vi "TURCK GUI TestPanel alle Module Test Lampe.vi"() -> ()   [LabVIEW 2017]
doc: "Example for reading and writing values for the TBEN-S2-2RFID-4DXP module from Turck"
uses:
  KH TURCK ETHERNETIP TDef Enum RFID Error.ctl
  KH TURCK ETHERNETIP TDefCluster TBEN-S2-2RFID-4DXP Status.ctl
  KH EthernetIPConfig 17.14/KH EthernetIPConfig TDef Config.ctl
  KH EthernetIPConfig 17.14/KH EthernetIPConfig TypeDefs ModuleTyp.ctl
  KH_DAQ 17.04/Turck/KH_DAQ_TURCK_TypeDefs_Cluster DI.ctl
  KH_DAQ 17.04/KH_DAQ_TypeDefs_Cluster AO.ctl
  KH_DAQ 17.04/KH_DAQ_TypeDefs_Messbereich.ctl
  KH_DAQ 17.04/KH_DAQ_TypeDefs_Bereich.ctl
  KH_DAQ 17.04/KH_DAQ_TypeDefs_Cluster AI.ctl
  KH TURCK ETHERNETIP TDef Enum IOL Data.ctl
  KH_DAQ 17.04/Turck/KH_DAQ_TURCK_TypeDefs_Cluster DO.ctl
  KH TURCK ETHERNETIP TDef Enum RFID Data RFID.ctl
  KH TURCK TypeDefs FGlob.ctl
  KH TURCK ETHERNETIP TDef Enum RFID User Command.ctl
  KH EthernetIP 17.19/KH_EthernetIP_Globals.vi
  KH TURCK ETHERNETIP RFID Global.vi
  KH TURCK ETHERNETIP RFID ST READ Global.vi
  KH TURCK ETHERNETIP Global.vi
panel:
  in  "Reset 7":bool
  in  "Reset 6":bool
  in  "Reset 5":bool
  in  "Reset 4":bool
  in  "Reset 3":bool
  in  "Reset 2":bool
  in  "Reset 1":bool
  in  "Reset 0":bool
  in  "Signal Name":string[](array[string])=["IOL1", "IOL3", "ARFID2", "ARFID3", "BRFID0", "BRFID1", "ADXP0", "ADXP2", "ADXP6", "ADXP7", "BDXP1", "BDXP2", "BDXP3", "BDXP7"]
  in  "DI":string[](array[string])=["IOL0", "IOL2", "ARFID0", "ARFID1", "BRFID2", "BRFID3", "ADXP1", "ADXP3", "ADXP4", "ADXP5", "BDXP0", "BDXP4", "BDXP5", "BDXP6"]
  out "DO in":bool[](array[boolean])
  out "DI":bool[](array[boolean])
  in  "AO Values":sgl[](array[numeric])=[0.0, 0.0, 0.0, 0.0, 0.0, 0.0, 0.0, 0.0] format="%.6f"
  in  "DO":bool[](array[boolean])=[FALSE, FALSE, FALSE, FALSE, FALSE, FALSE, FALSE, FALSE, FALSE, FALSE, FALSE, FALSE, FALSE, FALSE]
  in  "Tab Control":T1(tab)
  in  "EIP_DO":T2={"Def"=[], "Signal Name"=["IOL1", "IOL3", "ARFID2", "ARFID3", "BRFID0", "BRFID1", "ADXP0", "ADXP2", "ADXP6", "ADXP7", "BDXP1", "BDXP2", "BDXP3", "BDXP7"], "Description"=[], "Chan"=[], "Inv"=[], "Nr"=[1, 1, 1, 1, 2, 2, 1, 1, 1, 1, 2, 2, 2, 2], "SensorType"=[enum."TBEN-S2-4IOL", enum."TBEN-S2-4IOL", enum."TBEN-S2-2RFID-4DXP", enum."TBEN-S2-2RFID-4DXP", enum."TBEN-S2-2RFID-4DXP", enum."TBEN-S2-2RFID-4DXP", enum."TBEN-S1-8DXP", enum."TBEN-S1-8DXP", enum."TBEN-S1-8DXP", enum."TBEN-S1-8DXP", enum."TBEN-S1-8DXP", enum."TBEN-S1-8DXP", enum."TBEN-S1-8DXP", enum."TBEN-S1-8DXP"]} {"Nr" max=63; "Chan" max=63}
  in  "EIP_DI":T4={"Signal Name"=["IOL0", "IOL2", "ARFID0", "ARFID1", "BRFID2", "BRFID3", "ADXP1", "ADXP3", "ADXP4", "ADXP5", "BDXP0", "BDXP4", "BDXP5", "BDXP6"], "Description"=[], "Chan"=[], "Inv"=[], "Nr"=[1, 1, 1, 1, 2, 2, 1, 1, 1, 1, 2, 2, 2, 2], "SensorType"=[enum."TBEN-S2-4IOL", enum."TBEN-S2-4IOL", enum."TBEN-S2-2RFID-4DXP", enum."TBEN-S2-2RFID-4DXP", enum."TBEN-S2-2RFID-4DXP", enum."TBEN-S2-2RFID-4DXP", enum."TBEN-S1-8DXP", enum."TBEN-S1-8DXP", enum."TBEN-S1-8DXP", enum."TBEN-S1-8DXP", enum."TBEN-S1-8DXP", enum."TBEN-S1-8DXP", enum."TBEN-S1-8DXP", enum."TBEN-S1-8DXP"]} {"Nr" max=63; "Chan" max=63}
  in  "EIP_AO":T5={"Signal Name"=["AO0 Modul1", "AO1 Modul1", "AO2 Modul1", "AO3 Modul1", "AO0 Modul2", "AO1 Modul2", "AO2 Modul2", "AO3 Modul2"], "Description"=[], "Phys Unit"=[], "Messbereich"=[enum."0V ... +10V", enum."0V ... +10V", enum."0V ... +10V", enum."0V ... +10V", enum."0V ... +10V", enum."0V ... +10V", enum."0V ... +10V", enum."0V ... +10V"], "Chan"=[], "Phys Min"=[0.0, 0.0, 0.0, 0.0, 0.0, 0.0, 0.0, 0.0], "Phys Max"=[10.0, 10.0, 10.0, 10.0, 10.0, 10.0, 10.0, 10.0], "Offset"=[], "Nr"=[], "SensorType 2"=[enum."TBEN-S2-4AO", enum."TBEN-S2-4AO", enum."TBEN-S2-4AO", enum."TBEN-S2-4AO", enum."TBEN-S2-4AO", enum."TBEN-S2-4AO", enum."TBEN-S2-4AO", enum."TBEN-S2-4AO"], "Bereich"=[enum."Standard", enum."Standard", enum."Standard", enum."Standard", enum."Standard", enum."Standard", enum."Standard", enum."Standard"], "Default"=[]} {"Offset" format="%.4f"; "Phys Max" format="%.4f"; "Phys Min" format="%.4f"}
  in  "EIP_AI":T8={"Signal Name"=["AI0 Modul 1", "AI1 Modul 1", "AI2 Modul 1", "AI3 Modul 1", "AI0 Modul 2", "AI1 Modul 2", "AI2 Modul 2", "AI3 Modul 2"], "Description"=[], "Phys Unit"=[], "Messbereich"=[enum."0 Ohm ... 4000 Ohm", enum."0 Ohm ... 4000 Ohm", enum."0 Ohm ... 4000 Ohm", enum."0 Ohm ... 4000 Ohm", enum."0 Ohm ... 4000 Ohm", enum."0 Ohm ... 4000 Ohm", enum."0 Ohm ... 4000 Ohm", enum."0 Ohm ... 4000 Ohm"], "Chan"=[], "Phys Min"=[0.0, 0.0, 0.0, 0.0, 0.0, 0.0, 0.0, 0.0], "Phys Max"=[10.0, 10.0, 10.0, 10.0, 10.0, 10.0, 10.0, 10.0], "Offset"=[], "Nr"=[], "SensorType 2"=[enum."TBEN-S2-4AI", enum."TBEN-S2-4AI", enum."TBEN-S2-4AI", enum."TBEN-S2-4AI", enum."TBEN-S2-4AI", enum."TBEN-S2-4AI", enum."TBEN-S2-4AI", enum."TBEN-S2-4AI"], "Bereich"=[enum."Standard", enum."Standard", enum."Standard", enum."Standard", enum."Standard", enum."Standard", enum."Standard", enum."Standard"]} {"Offset" format="%.4f"; "Phys Max" format="%.4f"; "Phys Min" format="%.4f"}
  in  "Config File":path=path "C:/LabView/Kirschenhofer/EIP/KH Turck EthernetIP 17.12/examples/ini alle Module 10.ini"
  in  "Parameter RFID Array":T9(array[cluster])=[{"NumberOfBytes0"=312, "SizeFragmentRead1"=128, "SizeFragmentRead0"=128, "SizeFragmentWrite0"=128, "SizeFragmentWrite1"=128, "NumberOfBytes1"=312}, {"NumberOfBytes0"=312, "SizeFragmentRead1"=128, "SizeFragmentRead0"=128, "SizeFragmentWrite0"=128, "SizeFragmentWrite1"=128, "NumberOfBytes1"=312}]
  in  "Config":T10[](array[typedef])=[{"Typ"=enum."TBEN-S2-4IOL", "Name"="1", "Nr."=1, "InputOutput"=[enum."Input", enum."Output", enum."Input", enum."Output"]}, {"Typ"=enum."TBEN-S2-4AO", "Name"="2", "Nr."=1, "InputOutput"=[enum."Output", enum."Output", enum."Output", enum."Output"]}, {"Typ"=enum."TBEN-S2-4AO", "Name"="", "Nr."=2, "InputOutput"=[enum."Output", enum."Output", enum."Output", enum."Output"]}, {"Typ"=enum."TBEN-S2-2RFID-4DXP", "Name"="", "Nr."=1, "InputOutput"=[enum."Input", enum."Input", enum."Output", enum."Output"]}, {"Typ"=enum."TBEN-S2-2RFID-4DXP", "Name"="", "Nr."=2, "InputOutput"=[enum."Output", enum."Output", enum."Input", enum."Input"]}, {"Typ"=enum."TBEN-S1-8DXP", "Name"="", "Nr."=1, "InputOutput"=[enum."Output", enum."Input", enum."Output", enum."Input", enum."Input", enum."Input", enum."Output", enum."Output"]}, {"Typ"=enum."TBEN-S1-8DXP", "Name"="", "Nr."=2, "InputOutput"=[enum."Input", enum."Output", enum."Output", enum."Output", enum."Input", enum."Input", enum."Input", enum."Output"]}, {"Typ"=enum."TBEN-S2-4AI", "Name"="", "Nr."=1, "InputOutput"=[enum."Input", enum."Input", enum."Input", enum."Input"]}, {"Typ"=enum."TBEN-S2-4AI", "Name"="", "Nr."=2, "InputOutput"=[enum."Input", enum."Input", enum."Input", enum."Input"]}]
  in  "Write Kanal 0 Modul 1":u8[](array[numeric])
  in  "Write Kanal 1 Modul 1":u8[](array[numeric])
  in  "Write Kanal 0 Modul 2":u8[](array[numeric])
  in  "Write Kanal 1 Modul 2":u8[](array[numeric])
  out "Kanal 0 Modul 1":u8[](array[numeric])
  out "Kanal 0 Modul 2":u8[](array[numeric])
  out "Kanal 1 Modul 2":u8[](array[numeric])
  out "Kanal 1 Modul 1":u8[](array[numeric])
  out "UID Kanal 1 Modul 1":u8[](array[numeric])
  out "UID Kanal 1 Modul 2":u8[](array[numeric])
  out "UID Kanal 0 Modul2":u8[](array[numeric])
  out "UID Kanal 0 Modul 1":u8[](array[numeric])
  out "Error0 Modul 1":T11=33282
  out "Error1 Modul 1":T11=33282
  out "Error1 Modul 2":T11=33282
  out "Error0 Modul 2":T11=33282
  in  "Read":bool[](array[boolean])
  in  "Write":bool[](array[boolean])
  in  "Inventory":bool[](array[boolean])
  in  "Reset message":bool caption="Button"
  in  "TagNr":enum16{"Tag 0", "Tag 1"}(ring)
  out "Status Array":T12[](array[typedef])=[{"Error writing 1"=FALSE, "ReadingFinished 1"=FALSE, "WritingFinished 1"=FALSE, "Error writing 0"=FALSE, "ReadingFinished 0"=FALSE, "WritingFinished 0"=FALSE, "Timeout 1"=FALSE, "State0"="Idle", "State1"="Start", "Timeout 0"=FALSE, "Successfull Writing 1"=FALSE, "Successfull Writing 0"=FALSE}, {"Error writing 1"=FALSE, "ReadingFinished 1"=FALSE, "WritingFinished 1"=FALSE, "Error writing 0"=FALSE, "ReadingFinished 0"=FALSE, "WritingFinished 0"=FALSE, "Timeout 1"=TRUE, "State0"="", "State1"="", "Timeout 0"=FALSE, "Successfull Writing 1"=FALSE, "Successfull Writing 0"=FALSE}]
  out "RFID 0 Read SM":T13[](array[typedef])
  out "RFID 1 Read SM":T13[](array[typedef])
  out "DXP2":bool[](array[boolean])
  in  "DXP Status":string[](array[string])=["Channel 0 - Overcurrent", "Channel 1 - Overcurrent", "Channel 2 - Overcurrent", "Channel 3 - Overcurrent", "Channel 4 - Overcurrent", "Channel 5 - Overcurrent", "Channel 6 - Overcurrent", "Channel 7 - Overcurrent", "Overcurrent VAUX1 Ch0-3", "Overcurrent VAUX2 Ch4-7", "Channel 0 - Latch input", "Channel 1 - Latch input", "Channel 2 - Latch input", "Channel 3 - Latch input", "Channel 4 - Latch input", "Channel 5 - Latch input", "Channel 6 - Latch input", "Channel 7 - Latch input", "Module Diagnostics Available", "INFO: ARGEE Project Running", "Undervoltage V2", "Undervoltage V1", "Force Mode Enabled"]
  out "DXP1":bool[](array[boolean])
  out "AI2":bool[](array[boolean])
  in  "AI Status":string[](array[string])=["upper limit CH0", "upper limit CH1", "upper limit CH2", "upper limit CH3", "Overflow CH0", "Overflow CH1", "Overflow CH2", "Overflow CH3", "Underflow CH0", "Underflow CH1", "Underflow CH2", "Underflow CH3", "CJC Wire Break CH0", "CJC Wire Break CH1", "CJC Wire Break CH2", "CJC Wire Break CH3", "Overcurrent (RTD) CH0", "Overcurrent (RTD) CH1", "Overcurrent (RTD) CH2", "Overcurrent (RTD) CH3", "Wire break CH0", "Wire break CH1", "Wire break CH2", "Wire break CH3", "Overcurrent supply VAUX1 CH0", "Overcurrent supply VAUX1 CH1", "Overcurrent supply VAUX1 CH2", "Overcurrent supply VAUX1 CH3", "Lower limit value underrun CH0", "Lower limit value underrun CH1", "Lower limit value underrun CH2", "Lower limit value underrun CH3", "Module Diagnostics Available", "INFO: ARGEE Project Running", "Undervoltage Field Supply V2", "Undervoltage Field Supply V1", "Internal Error", "Force Mode Enabled"]
  out "AI":sgl[](array[numeric]) format="%.6f"
  out "AI1":bool[](array[boolean])
  in  "AO Status":string[](array[string])=["Modul 1 Overload Ch0", "Modul 1 Overload Ch1", "Modul 1 Overload Ch2", "Modul 1 Overload Ch3", "Modul 1 Wirebreak Ch0", "Modul 1 Wirebreak Ch1", "Modul 1 Wirebreak Ch2", "Modul 1 Wirebreak Ch3", "Modul 1 Module Diagnostics Available", "Modul 1 INFO: ARGEE Project Running", "Modul 1 Undervoltage V2", "Modul 1 Undervoltage V1", "Modul 1 Internal Error", "Modul 1 Force Mode Enabled", "Modul 2 Overload Ch0", "Modul 2 Overload Ch1", "Modul 2 Overload Ch2", "Modul 2 Overload Ch3", "Modul 2 Wirebreak Ch0", "Modul 2 Wirebreak Ch1", "Modul 2 Wirebreak Ch2", "Modul 2 Wirebreak Ch3", "Modul 2 Module Diagnostics Available", "Modul 2 INFO: ARGEE Project Running", "Modul 2 Undervoltage V2", "Modul 2 Undervoltage V1", "Modul 2 Internal Error", "Modul 2 Force Mode Enabled"]
  out "AO Status":bool[](array[boolean])
  in  "Output_IOL":T14={"IOL Port 1"=[0, 0], "IOL Port 2"=[0, 0], "IOL Port 3"=[0, 0], "IOL Port 4"=[0, 0]}
  out "IOL":T15
  out "error out":errorcluster
  in  "Exit":bool
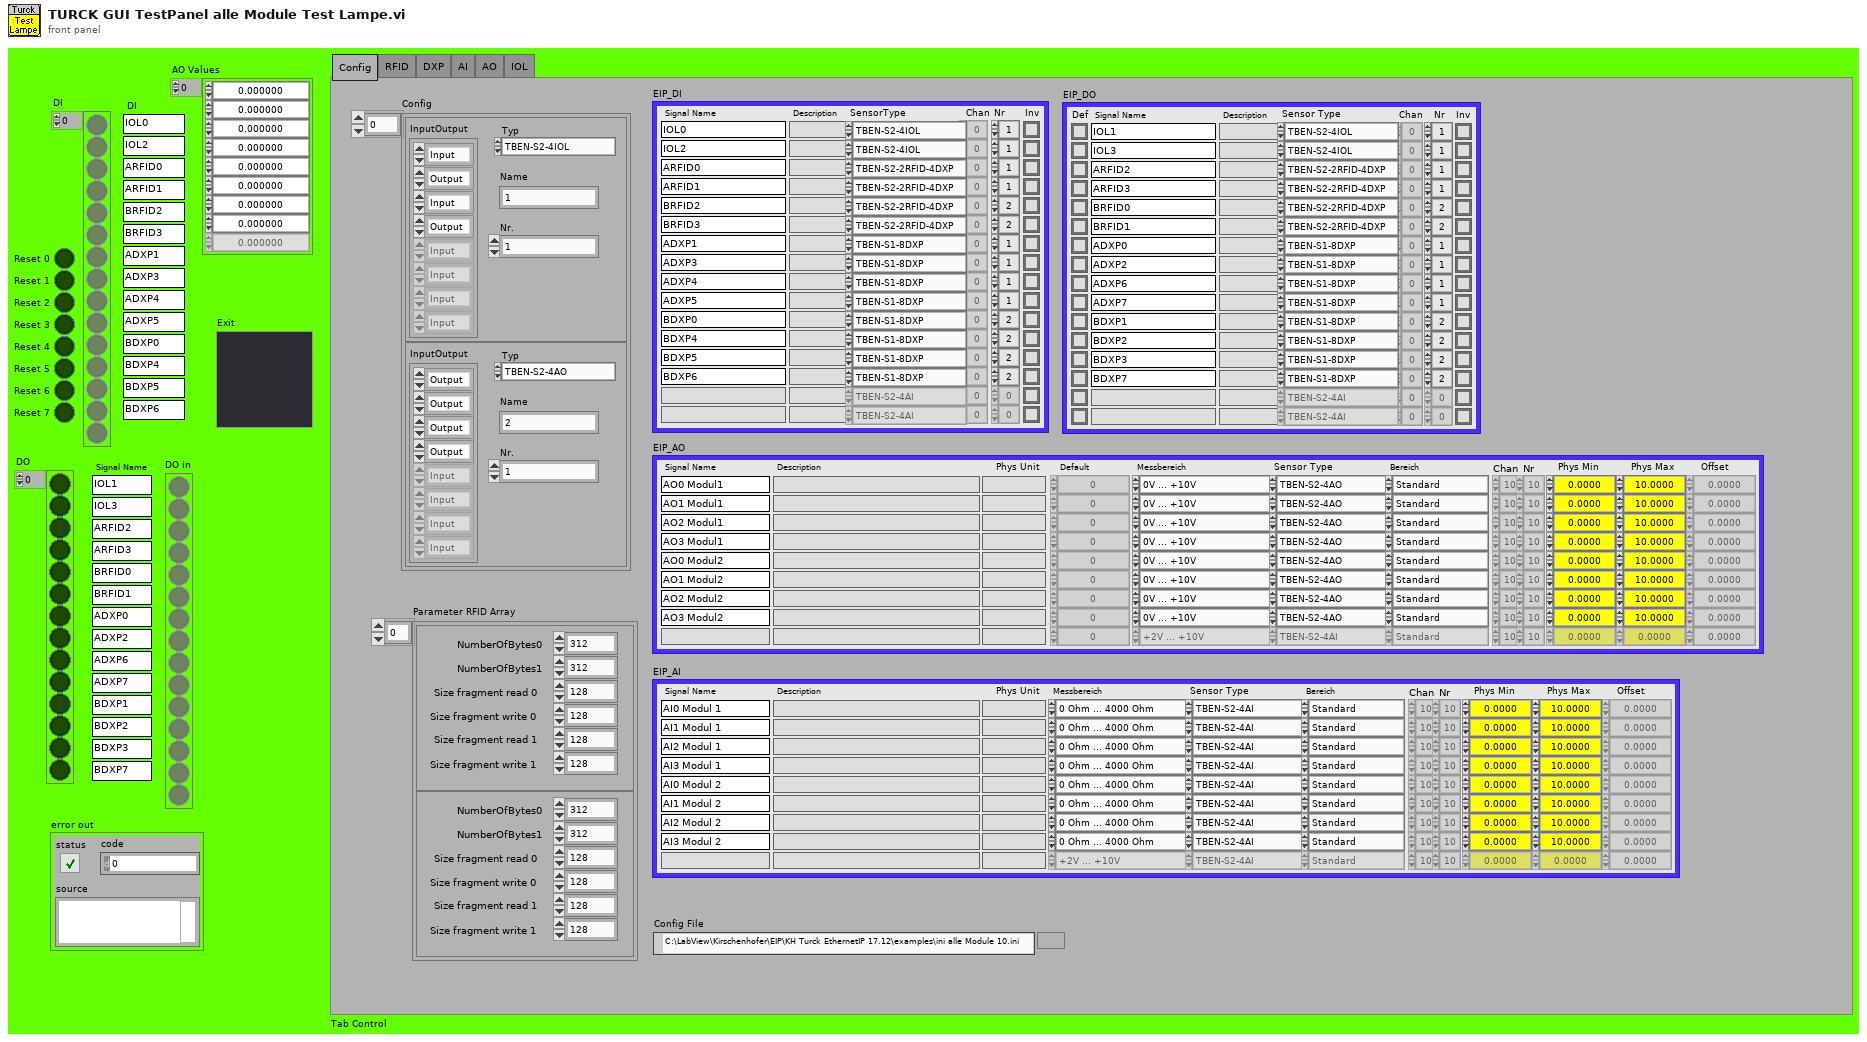
[diagram p1: front panel]
types:
  T1 = enum32{"Config", "RFID", "DXP", "AI", "AO", "IOL"}
  T2 = typedef "KH_DAQ_TURCK_TypeDefs_Cluster DO.ctl" = cluster{"Def":bool[], "Signal Name":string[], "Description":string[], "Chan":u16[], "Inv":bool[], "Nr":u16[], "SensorType":T3[]}
  T3 = typedef "KH EthernetIPConfig TypeDefs ModuleTyp.ctl" = enum16{"TBEN-S2-4AI", "TBEN-S1-8DXP", "TBEN-S2-2RFID-4DXP", "TBEN-S2-4AO", "TBEN-S2-4IOL"}
  T4 = typedef "KH_DAQ_TURCK_TypeDefs_Cluster DI.ctl" = cluster{"Signal Name":string[], "Description":string[], "Chan":u16[], "Inv":bool[], "Nr":u16[], "SensorType":T3[]}
  T5 = typedef "KH_DAQ_TypeDefs_Cluster AO.ctl" = cluster{"Signal Name":string[], "Description":string[], "Phys Unit":string[], "Messbereich":T6[], "Chan":u16[], "Phys Min":sgl[], "Phys Max":sgl[], "Offset":sgl[], "Nr":u16[], "SensorType 2":T3[], "Bereich":T7[], "Default":sgl[]}
  T6 = typedef "KH_DAQ_TypeDefs_Messbereich.ctl" = enum16{"-10V ... +10V", "0V ... +10V", "+2V ... +10V", "0V ... +5V", "+1V ... +5V", "-1V ... +1V", "-500mV ... +500mV", "-100mV ... +100mV", "-50mV ... +50mV", "0mA ... +20mA", "+4mA ... +20mA", "-20mA ... +20mA", "0 Ohm ... 100 Ohm", "0 Ohm ... 400 Ohm", "0 Ohm ... 2000 Ohm", "0 Ohm ... 4000 Ohm", "-200°C ... 150°C PT100", "-200°C ... 150°C PT200", "-200°C ... 150°C PT500", "-200°C ... 150°C PT1000", "-60°C ... 150°C Ni100", "-60°C ... 150°C Ni1000", "-200°C ... 850°C PT100", "-200°C ... 850°C PT200", "-200°C ... 850°C PT500", "-200°C ... 850°C PT1000", "-50°C ... 250°C Ni100", "-50°C ... 250° Ni 1000"}
  T7 = typedef "KH_DAQ_TypeDefs_Bereich.ctl" = enum16{"Standard", "extended Range", "NE43", ""}
  T8 = typedef "KH_DAQ_TypeDefs_Cluster AI.ctl" = cluster{"Signal Name":string[], "Description":string[], "Phys Unit":string[], "Messbereich":T6[], "Chan":u16[], "Phys Min":sgl[], "Phys Max":sgl[], "Offset":sgl[], "Nr":u16[], "SensorType 2":T3[], "Bereich":T7[]}
  T9 = cluster{"NumberOfBytes0":i32, "SizeFragmentRead1":i32, "SizeFragmentRead0":i32, "SizeFragmentWrite0":i32, "SizeFragmentWrite1":i32, "NumberOfBytes1":i32}[]
  T10 = typedef "KH EthernetIPConfig TDef Config.ctl" = cluster{"Typ":T3, "Name":string, "Nr.":i32, "InputOutput":enum16{"Input", "Output"}[]}
  T11 = typedef "KH TURCK ETHERNETIP TDef Enum RFID Error.ctl" = u16
  T12 = typedef "KH TURCK ETHERNETIP TDefCluster TBEN-S2-2RFID-4DXP Status.ctl" = cluster{"Error writing 1":bool, "ReadingFinished 1":bool, "WritingFinished 1":bool, "Error writing 0":bool, "ReadingFinished 0":bool, "WritingFinished 0":bool, "Timeout 1":bool, "State0":string, "State1":string, "Timeout 0":bool, "Successfull Writing 1":bool, "Successfull Writing 0":bool}
  T13 = typedef "KH TURCK ETHERNETIP TDef Enum RFID Data RFID.ctl" = cluster{"ResponseCode":u16, "LoopCounter":u8, "Length":u16, "WriteFragmentNo":u8, "ReadFragmentNo":u8, "Data":u8[], "TagPresent":bool, "Error":bool, "BusyFinished":bool, "Channel":u16}
  T14 = cluster{"IOL Port 1":u16[], "IOL Port 2":u16[], "IOL Port 3":u16[], "IOL Port 4":u16[]}
  T15 = typedef "KH TURCK ETHERNETIP TDef Enum IOL Data.ctl" = cluster{"Data_Port1":u16[], "Data_Port3":u16[], "Data_Port5":u16[], "Data_Port7":u16[], "Status":cluster{"Undervoltage Field Supply V2":bool, "Overvoltage Field Supply V1":bool, "Undervoltage Field Supply V1":bool, "Internal Error":bool, "Module Diagnostics Available":bool, "Station Configuration Changed":bool, "Overcurrent Isys":bool, "Overvoltage Field Supply V2":bool, "Force Mode Enabled":bool}, "Diagnostics":cluster{"Channel 2 - Output signal overcurrent":bool, "Channel 4 - Output signal overcurrent":bool, "Channel 6 - Output signal overcurrent":bool, "Channel 8 - Output signal overcurrent":bool, "Channel 1 - Wrong or missing device":bool, "Channel 3 - Wrong or missing device":bool, "Channel 5 - Wrong or missing device":bool, "Channel 7 - Wrong or missing device":bool, "Channel 1 - Data storage error":bool, "Channel 3 - Data storage error":bool, "Channel 5 - Data storage error":bool, "Channel 7 - Data storage error":bool, "Channel 1 - Process input data invalid":bool, "Channel 3 - Process input data invalid":bool, "Channel 5 - Process input data invalid":bool, "Channel 7 - Process input data invalid":bool, "Channel 1 - Hardware error":bool, "Channel 3 - Hardware error":bool, "Channel 5 - Hardware error":bool, "Channel 7 - Hardware error":bool, "Channel 1 - Maintenance events":bool, "Channel 3 - Maintenance events":bool, "Channel 5 - Maintenance events":bool, "Channel 7 - Maintenance events":bool, "Channel 1 - Out of spec. error":bool, "Channel 3 - Out of spec. error":bool, "Channel 5 - Out of spec. error":bool, "Channel 7 - Out of spec. error":bool, "Channel 1 - Parameterization error":bool, "Channel 3 - Parameterization error":bool, "Channel 5 - Parameterization error":bool, "Channel 1 - Overtemperature":bool, "Channel 3 - Overtemperature":bool, "Channel 5 - Overtemperature":bool, "Channel 7 - Overtemperature":bool, "Channel 1 - Lower limit value underrun":bool, "Channel 3 - Lower limit value underrun":bool, "Channel 5 - Lower limit value underrun":bool, "Channel 7 - Lower limit value underrun":bool, "Channel 1 - Upper limit value exceeded":bool, "Channel 3 - Upper limit value exceeded":bool, "Channel 5 - Upper limit value exceeded":bool, "Channel 7 - Upper limit value exceeded":bool, "Channel 1 - Undervoltage":bool, "Channel 3 - Undervoltage":bool, "Channel 5 - Undervoltage":bool, "Channel 7 - Undervoltage":bool, "Channel 1 - Overvoltage":bool, "Channel 3 - Overvoltage":bool, "Channel 5 - Overvoltage":bool, "Channel 7 - Overvoltage":bool, "Channel 1 - Overload":bool, "Channel 3 - Overload":bool, "Channel 5 - Overload":bool, "Channel 7 - Overload":bool, "Channel 1 - Common error":bool, "Channel 3 - Common error":bool, "Channel 5 - Common error":bool, "Channel 7 - Common error":bool, "Channel 1 - Port parameterization error":bool, "Channel 3 - Port parameterization error":bool, "Channel 5 - Port parameterization error":bool, "Channel 7 - Parameterization error":bool, "Channel 7 - Port parameterization error":bool}, "Events":cluster{"Event":u8[], "Qualifier":u8[], " Event code":u16[]}, "DXP":cluster{"DI Input value 2":bool, "DI Input value 4":bool, "DI Input value 6":bool, "DI Input value 8":bool, "DI Input 1":bool, "DI Input 3":bool, "DI Input 5":bool, "DI Input 7":bool, "Input values valid 1":bool, "Input values valid 3":bool, "Input values valid 5":bool, "Input values valid 7":bool}}
  T16 = typedef "KH TURCK TypeDefs FGlob.ctl" = enum16{"Put one", "Put all", "Recall one", "Recall all"}
  T17 = typedef "KH TURCK ETHERNETIP TDef Enum RFID User Command.ctl" = enum16{"read", "write", "idle", "inventory"}
  T18 = typedef "KH TURCK ETHERNETIP TDefCluster TURCK RFID.ctl" = cluster{"NumberOfBytes":i32, "State":string, "Counter":i32, "ReadData":u8[], "AnzahlFragmente":i32, "WritingFinished":bool, "ReadingFinished":bool, "UID":u8[], "ActCommand":T19, "SizeFragmentRead":i32, "LengthUID":u16, "WriteDataInclUID":u8[], "Timeout":bool, "SizeFragmentWrite":i32}
  T19 = typedef "KH TURCK ETHERNETIP TDef Enum RFID Act Command.ctl" = enum16{"read", "write", "idle", "Inventory", ""}
  T20 = typedef "KH TURCK ETHERNETIP TDefCluster TBEN-S2-2RFID-4DXP Input Values.ctl" = cluster{"Station Status Word (Input Data Mapping)":cluster{"Module diagnostics avaliable":bool, "INFO: ARGEE Project Running":bool, "Undervoltage V2":bool, "Undervoltage V1":bool, "Internal Error":bool, "I/O-ASSISTANT Force Mode active":bool}, "RFID control/status 0 (Input Data Mapping)":cluster{"Tag present at r/w head":bool[], "response code":u16, "loop counter":u8, "Length":u16, "Error code":u16, "Tag counter":u16, "Data (Bytes) available":u16, "Read fragment No.":u8, "Write fragment No.":u8, "Tag present at r/w head bit":bool, "HF r/w head switched on":bool, "Continuous mode active":bool, "Antenna detuned at HF read/write head":bool, "Parameter not supported by read/write head":bool, "Error reported by read/write head":bool, "Not connected to read/write head":bool}, "RFID read data 0 (Input Data Mapping)":u8[], "RFID control/status 1 (Input Data Mapping)":cluster{"response code":u16, "Loop counter":u8, "Length":u16, "Error code":u16, "Tag counter":u16, "Data (Bytes) available":u16, "Read fragment No.":u8, "Write fragment No.":u8, "Tag present at r/w head bit":bool, "HF r/w head switched on":bool, "Continuous mode active":bool, "Antenna detuned at HF read/write head":bool, "Parameter not supported by read/write head":bool, "Error reported by read/write head":bool, "Not connected to read/write head":bool, "Tag present at r/w head":bool[]}, "RFID read data 1 (Input Data Mapping)":u8[], "RFID diagnostics (Input Data Mapping)":cluster{"Overcurrent supply VAUX1 (a)":bool, "Parameterization error (a)":bool, "Configuration via DTM active (a)":bool, "Buffer full (a)":bool, "Antenna detuned at HF read/write head (a)":bool[], "Parameter not supported by read/write head (a)":bool[], "Error reported by read/write head (a)":bool[], "Not connected to read/write head (a)":bool[], "Overcurrent supply VAUX1 (b)":bool, "Parameterization error (b)":bool, "Configuration via DTM active (b)":bool, "Buffer full (b)":bool, "Antenna detuned at HF read/write head (b)":bool[], "Parameter not supported by read/write head (b)":bool[], "Error reported by read/write head (b)":bool[], "Not connected to read/write head (b)":bool[]}, "DXP diagnostics (Input Data Mapping)":cluster{"Overcurrent VAUX2 Ch4/5":bool, "Overcurrent VAUX2 Ch6/7":bool, "Channel 4 - Output overcurrent":bool, "Channel 5 - Output overcurrent":bool, "Channel 6 - Output overcurrent":bool, "Channel 7 - Output overcurrent":bool}, "DXP (Input Data Mapping)":cluster{"Channel 4 - Input value":bool, "Channel 5 - Input value":bool, "Channel 6 - Input value":bool, "Channel 7 - Input value":bool}}
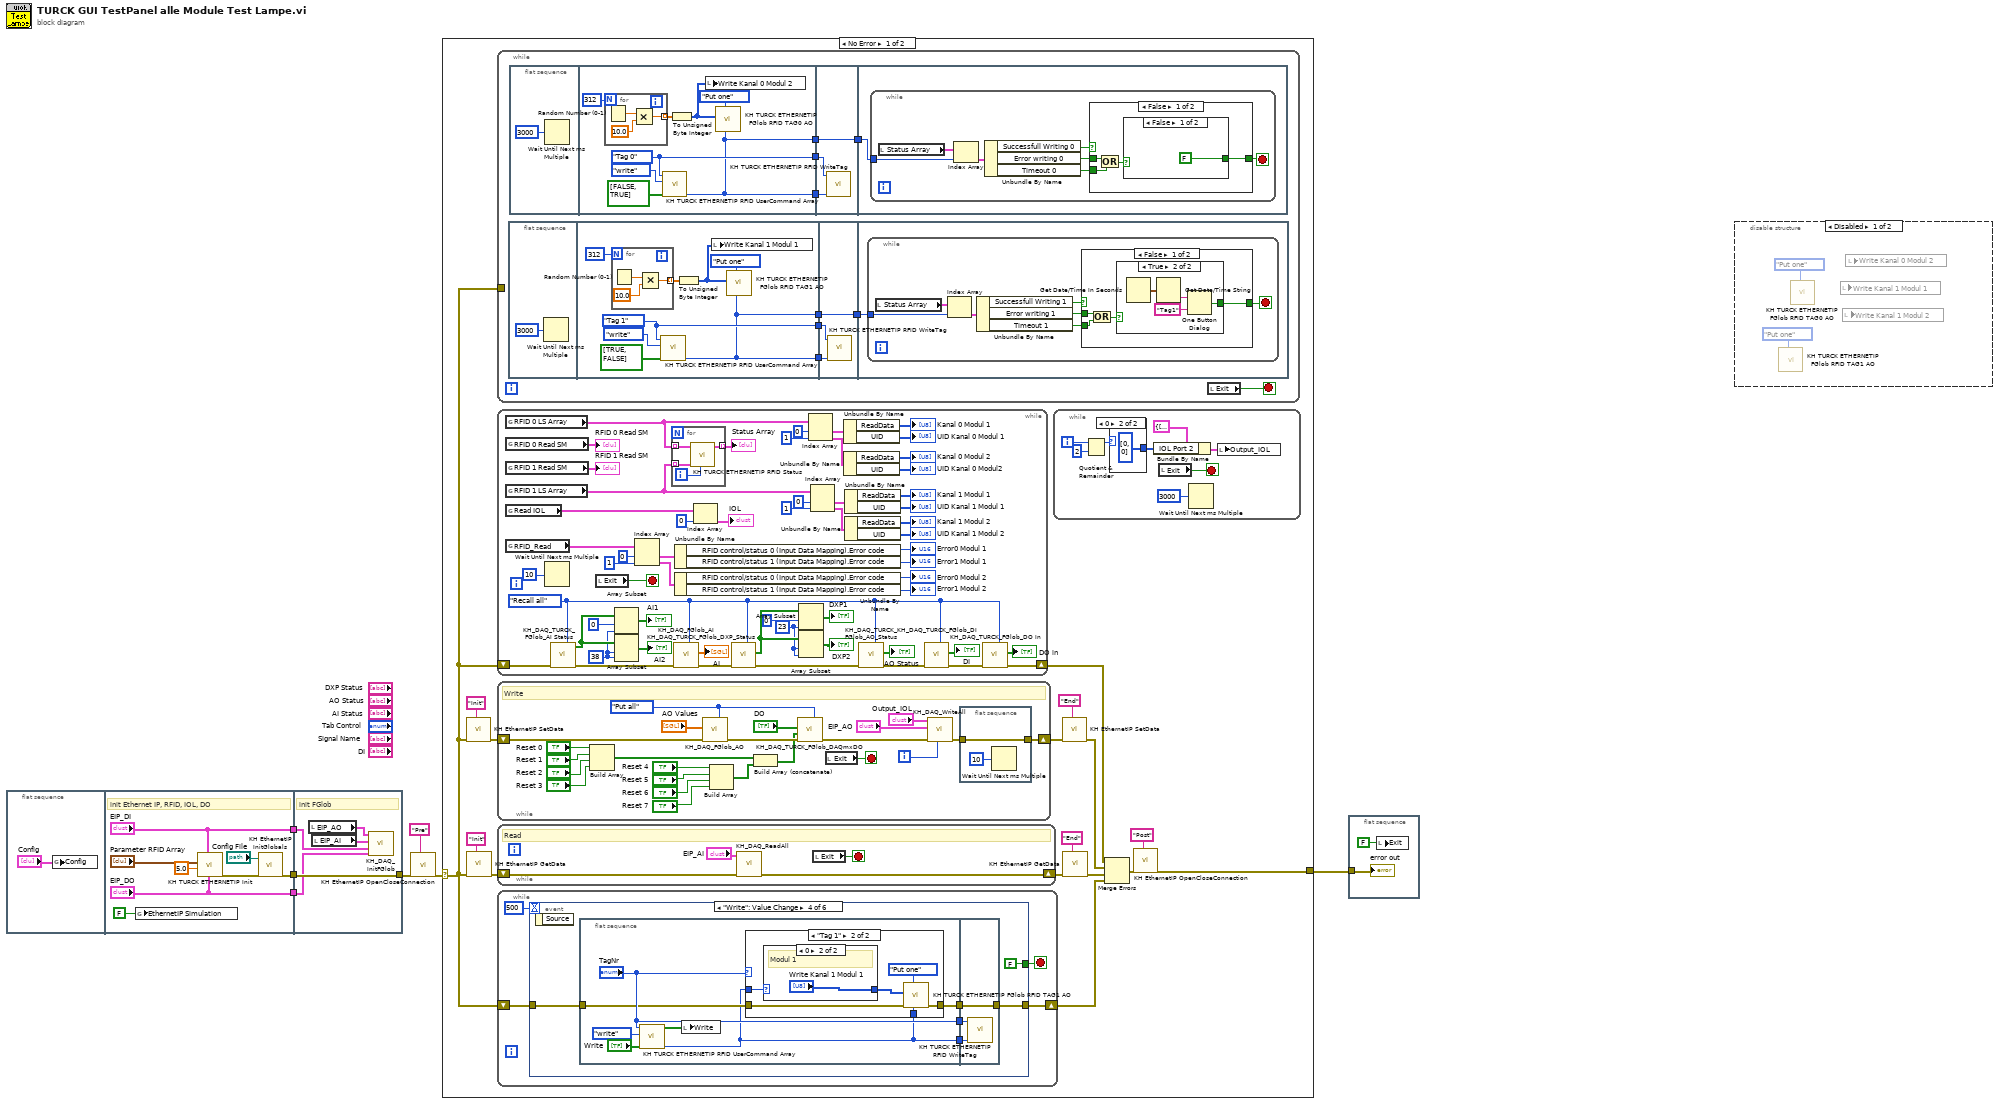
[diagram p0: block diagram]
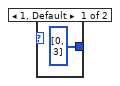
[diagram p3: hidden frame]
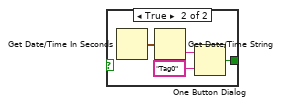
[diagram p4: hidden frame]
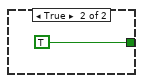
[diagram p5: hidden frame]
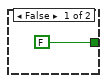
[diagram p6: hidden frame]
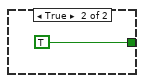
[diagram p7: hidden frame]
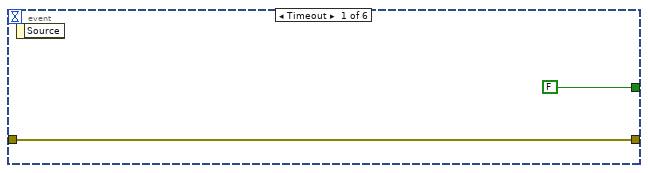
[diagram p8: hidden frame]
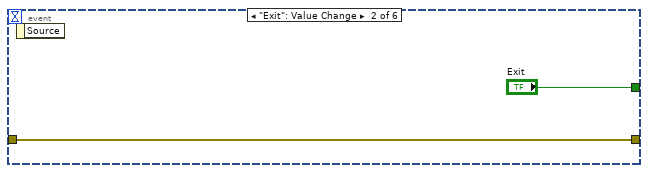
[diagram p9: hidden frame]
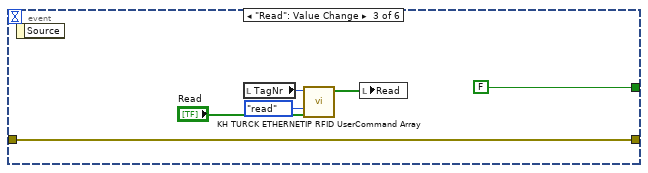
[diagram p10: hidden frame]
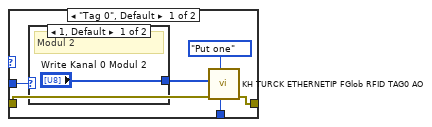
[diagram p11: hidden frame]
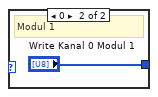
[diagram p12: hidden frame]
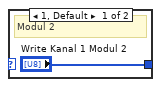
[diagram p13: hidden frame]
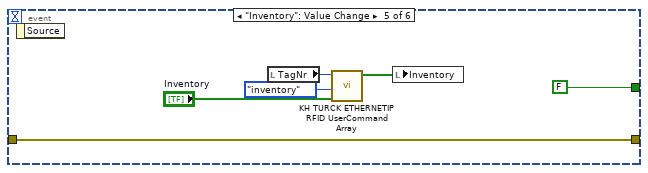
[diagram p14: hidden frame]
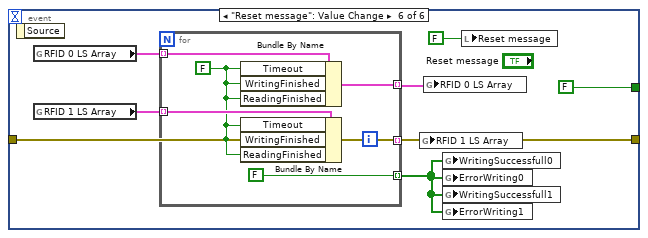
[diagram p15: hidden frame]
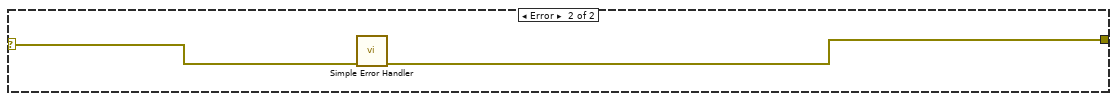
[diagram p16: hidden frame]
diagram:
  n1 = flat-sequence {
    tunnel: [w16] -> w3
    tunnel: ["EIP_DI"] -> w2
    tunnel: ["EIP_DO"] -> w1
    tunnel: [w19] -> w5
    tunnel: w3 -> [w19]
    tunnel: w2 -> [w18]
    tunnel: w1 -> [w17]
    frame #0 {
      n2 = global write "KH_EthernetIP_Globals.vi" "Config"("Config") -> ()
    }
    frame #1 {
      # "init Ethernet IP, RFID, IOL, DO"
      n3 = global write "KH_EthernetIP_Globals.vi" "EthernetIP Simulation"(FALSE ("EthernetIP Simulation")) -> ()
      n4 = call "KH TURCK ETHERNETIP Init.vi"("EIP_DO"="EIP_DO", "EIP_DI"="EIP_DI", "TimeoutRFID"=5.0 ("Timeout"), "Parameter RFID Array"="Parameter RFID Array") -> ("err out"=w12:errorcluster)  [unwired: 7 in]
      n5 = call "KH EthernetIP InitGlobals.vi"("err in"=w12, "Config File"="Config File") -> ("err out"=w16:errorcluster)  [unwired: 9 in]
    }
    frame #2 {
      # "init FGlob"
      n6 = local read "EIP_AO"() -> (w20:T5)
      n7 = local read "EIP_AI"() -> (w21:T8)
      n8 = call "KH_DAQ_InitFGlob.vi"("EIP_DO"=w17, "EIP_DI"=w18, "EIP_AI"=w21, "EIP_AO"=w20) -> ()  [unwired: 8 in]
    }
  }
  n9 = call "KH EthernetIP OpenCloseConnection.vi"("Function"="Pre", "error in"=w5) -> ("error out"=w6:errorcluster)  [unwired: 9 in]
  n10 = case shown="No Error" w6 {
    selector: w6 -> [w22 w280]
    tunnel: [w25 w279] -> w4
    frame No Error {
      n11 = call "KH EthernetIP SetData.vi"("Function"="Init", "error in"=w22) -> ("error out"=w24:errorcluster)  [unwired: 7 in, 2 out]
      n12 = call "KH EthernetIP GetData.vi"("Function"="Init", "error in"=w22) -> ("error out"=w37:errorcluster)  [unwired: 8 in, 1 out]
      n13 = while {
        tunnel: w22 -> [_]
        stop <- w56 stop-if-true
        n14 = flat-sequence {
          tunnel: [w94] -> w55
          tunnel: [w96] -> w54
          tunnel: [w94] -> w50
          tunnel: w55 -> [w104]
          tunnel: w54 -> [w103]
          tunnel: [w102] -> w51
          tunnel: w50 -> [w102]
          tunnel: w51 -> [w105]
          frame #0 {
            n15 = Wait Until Next ms Multiple(millisecond multiple=u32 3000) -> ()  [unwired: 1 out]
          }
          frame #1 {
            w96 = enum16{"Tag 0", "Tag 1"}."Tag 1" ("TagNr")
            n16 = for {
              N: 312 -> [_]
              tunnel: [w100] -> w92 mode=indexing
              n17 = Random Number (0-1)() -> (number: 0 to 1=w99:dbl)
              n18 = Multiply(x=w99, y=10.0) -> (x*y=w100:dbl)
            }
            n19 = call "KH TURCK ETHERNETIP RFID UserCommand Array.vi"("BitArray"=bool[] [TRUE, FALSE], "UserCommand"=KH_TURCK_ETHERNETIP_TDef_Enum_RFID_User_Command."write", "TagNr"=w96) -> ("index of element"=w94:i32)  [unwired: 7 in, 1 out]
            n20 = To Unsigned Byte Integer(number=w92) -> (unsigned 8bit integer=w91:u8[])
            n21 = local write "Write Kanal 1 Modul 1"(w91) -> ()
            n22 = call "KH TURCK ETHERNETIP FGlob RFID TAG1 AO.vi"("Nr Module"=w94, "Function"=KH_TURCK_TypeDefs_FGlob."Put one", "RFID one in"=w91) -> ()  [unwired: 6 in, 3 out]
          }
          frame #2 {
            n23 = call "KH TURCK ETHERNETIP RFID WriteTag.vi"("Modul Nr"=w104, "TagNr"=w103) -> ()  [unwired: 10 in]
          }
          frame #3 {
            n24 = while {
              tunnel: w105 -> [w107]
              stop <- w106 stop-if-true
              n25 = local read "Status Array"() -> (w112:T12[])
              n26 = Index Array(array=w112, index=w107) -> (element=w111:T12)
              n27 = Unbundle By Name(w111) -> ("Successfull Writing 1"=w110:bool, "Error writing 1"=w109:bool, "Timeout 1"=w108:bool)
              n28 = case shown="False" w110 {
                tunnel: [w113 TRUE] -> w106
                tunnel: w109 -> [w116 _]
                tunnel: w108 -> [w115 _]
                frame False {
                  n29 = Or(x=w116, y=w115) -> (x .or. y?=w114:bool)
                  n30 = case shown="True" w114 {
                    tunnel: [FALSE w118] -> w113
                    frame False {
                    }
                    frame True {
                      n31 = Get Date/Time In Seconds() -> (seconds since 1Jan1904=w121:timestamp)
                      n32 = Get Date/Time String(seconds (now)=w121) -> (time string=w120:string)  [unwired: 2 in, 1 out]
                      n33 = One Button Dialog(message=w120, button name ("OK")="Tag1") -> (true=w118:bool)
                    }
                  }
                }
                frame True {
                }
              }
            }
          }
        }
        n34 = flat-sequence {
          tunnel: [w59] -> w53
          tunnel: [w63] -> w52
          tunnel: [w59] -> w48
          tunnel: w53 -> [w71]
          tunnel: w52 -> [w70]
          tunnel: [w69] -> w49
          tunnel: w48 -> [w69]
          tunnel: w49 -> [w72]
          frame #0 {
            n35 = Wait Until Next ms Multiple(millisecond multiple=u32 3000) -> ()  [unwired: 1 out]
          }
          frame #1 {
            w63 = enum16{"Tag 0", "Tag 1"}."Tag 0" ("TagNr")
            n36 = for {
              N: 312 -> [_]
              tunnel: [w67] -> w60 mode=indexing
              n37 = Random Number (0-1)() -> (number: 0 to 1=w66:dbl)
              n38 = Multiply(x=w66, y=10.0) -> (x*y=w67:dbl)
            }
            n39 = call "KH TURCK ETHERNETIP RFID UserCommand Array.vi"("BitArray"=bool[] [FALSE, TRUE], "UserCommand"=KH_TURCK_ETHERNETIP_TDef_Enum_RFID_User_Command."write", "TagNr"=w63) -> ("index of element"=w59:i32)  [unwired: 7 in, 1 out]
            n40 = To Unsigned Byte Integer(number=w60) -> (unsigned 8bit integer=w58:u8[])
            n41 = local write "Write Kanal 0 Modul 2"(w58) -> ()
            n42 = call "KH TURCK ETHERNETIP FGlob RFID TAG0 AO.vi"("Nr Module"=w59, "Function"=KH_TURCK_TypeDefs_FGlob."Put one", "RFID one in"=w58) -> ()  [unwired: 6 in, 3 out]
          }
          frame #2 {
            n43 = call "KH TURCK ETHERNETIP RFID WriteTag.vi"("Modul Nr"=w71, "TagNr"=w70) -> ()  [unwired: 10 in]
          }
          frame #3 {
            n44 = while {
              tunnel: w72 -> [w74]
              stop <- w73 stop-if-true
              n45 = local read "Status Array"() -> (w79:T12[])
              n46 = Index Array(array=w79, index=w74) -> (element=w78:T12)
              n47 = Unbundle By Name(w78) -> ("Successfull Writing 0"=w77:bool, "Error writing 0"=w76:bool, "Timeout 0"=w75:bool)
              n48 = case shown="False" w77 {
                tunnel: w76 -> [w83 _]
                tunnel: w75 -> [w82 _]
                tunnel: [w80 TRUE] -> w73
                frame False {
                  n49 = Or(x=w83, y=w82) -> (x .or. y?=w81:bool)
                  n50 = case shown="False" w81 {
                    tunnel: [FALSE w85] -> w80
                    frame False {
                    }
                    frame True {
                      n51 = Get Date/Time In Seconds() -> (seconds since 1Jan1904=w88:timestamp)
                      n52 = Get Date/Time String(seconds (now)=w88) -> (time string=w87:string)  [unwired: 2 in, 1 out]
                      n53 = One Button Dialog(message=w87, button name ("OK")="Tag0") -> (true=w85:bool)
                    }
                  }
                }
                frame True {
                }
              }
            }
          }
        }
        n54 = local read "Exit"() -> (w56:bool)
      }
      n55 = while {
        shift-right: [w174] -> w23
        shift-left: w22 -> [w136]
        stop <- w173 stop-if-true
        w125 = 23 ("length")
        w142 = 38 ("index")
        w172 = KH_TURCK_TypeDefs_FGlob."Recall all" ("Function (Recall One)")
        n56 = global read "KH TURCK ETHERNETIP RFID Global.vi" "RFID 0 LS Array"() -> (w155:T18[])
        n57 = global read "KH TURCK ETHERNETIP RFID ST READ Global.vi" "RFID 0 Read SM"() -> (→"RFID 0 Read SM":T13[])
        n58 = global read "KH TURCK ETHERNETIP RFID ST READ Global.vi" "RFID 1 Read SM"() -> (→"RFID 1 Read SM":T13[])
        n59 = global read "KH TURCK ETHERNETIP RFID Global.vi" "RFID 1 LS Array"() -> (w161:T18[])
        n60 = global read "KH TURCK ETHERNETIP Global.vi" "Read IOL"() -> (w123:T15[])
        n61 = global read "KH TURCK ETHERNETIP Global.vi" "RFID_Read"() -> (w124:T20[])
        n62 = Wait Until Next ms Multiple(millisecond multiple=u32 10) -> ()  [unwired: 1 out]
        n63 = call "KH_DAQ_TURCK_FGlob_AI Status.vi"("Function (Recall One)"=w172, "err in"=w136) -> ("err out"=w179:errorcluster, "StatusOut"=w144:bool[])  [unwired: 7 in, 1 out]
        n64 = local read "Exit"() -> (w173:bool)
        n65 = Array Subset(array=w144, index=0, length=w142) -> (→"AI1":bool[])
        n66 = Array Subset(array=w144, index=w142, length=w142) -> (→"AI2":bool[])
        n67 = Index Array(array=w124, index #1=0 ("index"), index #2=1 ("index")) -> (element #1=w165:T20, element #2=w130:T20)
        n68 = for {
          tunnel: w155 -> [w183] mode=indexing
          tunnel: w161 -> [w182] mode=indexing
          tunnel: [w181] -> w150 mode=indexing
          i -> [w180]
          n69 = call "KH TURCK ETHERNETIP RFID Status.vi"("Nr.Module"=w180, "RFID 1"=w182, "RFID 0"=w183) -> ("StatusOUT"=w181:T12)  [unwired: 8 in]
        }
        "Status Array" <- w150
        n70 = call "KH_DAQ_FGlob_AI.vi"("Function (Recall One)"=w172, "err in"=w179) -> ("err out"=w178:errorcluster, "AI Values OUT"=→"AI":sgl[])  [unwired: 6 in, 2 out]
        n71 = Unbundle By Name(w165) -> ("RFID control/status 0 (Input Data Mapping).Error code"=→"Error0 Modul 1":u16, "RFID control/status 1 (Input Data Mapping).Error code"=→"Error1 Modul 1":u16)
        n72 = Unbundle By Name(w130) -> ("RFID control/status 0 (Input Data Mapping).Error code"=→"Error0 Modul 2":u16, "RFID control/status 1 (Input Data Mapping).Error code"=→"Error1 Modul 2":u16)
        n73 = Index Array(array=w123, index=0) -> (element=→"IOL":T15)
        n74 = call "KH_DAQ_TURCK_FGlob_DXP_Status.vi"("Function (Recall One)"=w172, "err in"=w178) -> ("err out"=w177:errorcluster, "DXP Status OUT"=w129:bool[])  [unwired: 8 in]
        n75 = Array Subset(array=w129, index=0, length=w125) -> (→"DXP1":bool[])
        n76 = Array Subset(array=w129, index=w125, length=w125) -> (→"DXP2":bool[])
        n77 = Index Array(array=w155, index #1=0 ("index"), index #2=1 ("index")) -> (element #1=w151:T18, element #2=w135:T18)
        n78 = Index Array(array=w161, index #1=0 ("index"), index #2=1 ("index")) -> (element #1=w159:T18, element #2=w132:T18)
        n79 = Unbundle By Name(w151) -> ("ReadData"=→"Kanal 0 Modul 1":u8[], "UID"=→"UID Kanal 0 Modul 1":u8[])
        n80 = Unbundle By Name(w135) -> ("ReadData"=→"Kanal 0 Modul 2":u8[], "UID"=→"UID Kanal 0 Modul2":u8[])
        n81 = Unbundle By Name(w159) -> ("ReadData"=→"Kanal 1 Modul 1":u8[], "UID"=→"UID Kanal 1 Modul 1":u8[])
        n82 = Unbundle By Name(w132) -> ("ReadData"=→"Kanal 1 Modul 2":u8[], "UID"=→"UID Kanal 1 Modul 2":u8[])
        n83 = call "KH_DAQ_TURCK_FGlob_AO_Status.vi"("Function (Recall One)"=w172, "err in"=w177) -> ("err out"=w176:errorcluster, "AO Status OUT"=→"AO Status":bool[])  [unwired: 8 in]
        n84 = call "KH_DAQ_TURCK_FGlob_DI.vi"("Function (Recall One)"=w172, "err in"=w176) -> ("err out"=w175:errorcluster, "DI Values OUT"=→"DI":bool[])  [unwired: 7 in, 1 out]
        n85 = call "KH_DAQ_TURCK_FGlob_DO In.vi"("Function (Recall One)"=w172, "err in"=w175) -> ("err out"=w174:errorcluster, "DO in Values OUT"=→"DO in":bool[])  [unwired: 7 in, 1 out]
      }
      n86 = while {
        shift-right: [w203] -> w28
        shift-left: w24 -> [w197]
        i -> [w202]
        stop <- w206 stop-if-true
        w198 = KH_TURCK_TypeDefs_FGlob."Put all" ("Function (Recall One)")
        # "Write"
        n87 = Build Array("Reset 0", "Reset 1", "Reset 2", "Reset 3") -> (w186:bool[])
        n88 = call "KH_DAQ_FGlob_AO.vi"("Function (Recall One)"=w198, "err in"=w197, "AO Values IN"="AO Values") -> ("err out"=w191:errorcluster)  [unwired: 6 in, 2 out]
        n89 = Build Array("Reset 4", "Reset 5", "Reset 6", "Reset 7") -> (w185:bool[])
        n90 = Build Array (concatenate)(w186, w185) -> (w184:bool[])
        n91 = call "KH_DAQ_TURCK_FGlob_DAQmxDO.vi"("Function (Recall One)"=w198, "err in"=w191, "DXP Reset IN"=w184, "DXP Values IN"="DO") -> ("err out"=w196:errorcluster)  [unwired: 4 in, 3 out]
        n92 = local read "Exit"() -> (w206:bool)
        n93 = call "KH_DAQ_WriteAll.vi"("Numeric"=w202, "err in"=w196, "EIP_AO"="EIP_AO", "Output_IOL"="Output_IOL") -> ("err out"=w204:errorcluster)  [unwired: 7 in]
        n94 = flat-sequence {
          tunnel: w204 -> [w207]
          tunnel: [w207] -> w203
          frame #0 {
            n95 = Wait Until Next ms Multiple(millisecond multiple=u32 10) -> ()  [unwired: 1 out]
          }
        }
      }
      n96 = while {
        shift-right: [w209] -> w35
        shift-left: w37 -> [w211]
        stop <- w212 stop-if-true
        # "Read"
        n97 = call "KH_DAQ_ReadAll.vi"("err in"=w211, "EIP_AI"="EIP_AI") -> ("err out"=w209:errorcluster)  [unwired: 9 in]
        n98 = local read "Exit"() -> (w212:bool)
      }
      n99 = while {
        shift-right: [w213] -> w26
        shift-left: w22 -> [w215]
        stop <- w216 stop-if-true
        n100 = event shown="[3] \"Write\": Value Change" {
          selector: _ -> [_ _ _ _ _ _]
          dyn-events: _ -> [_ _ _ _ _ _]
          timeout: 500 -> [_ _ _ _ _ _]
          tunnel: [FALSE ("Exit") "Exit" FALSE ("Exit") FALSE ("Exit") FALSE ("Exit") FALSE ("Exit")] -> w216
          tunnel: w215 -> [w217 w219 w225 w231 w263 w271]
          tunnel: [w217 w219 w225 w230 w263 w271] -> w213
          event Timeout {
            n101 = event-data() -> ()  [unwired: 1 in, 1 out]
          }
          event "Exit": Value Change {
            n102 = event-data() -> ()  [unwired: 1 in, 1 out]
          }
          event "Read": Value Change {
            n103 = event-data() -> ()  [unwired: 1 in, 1 out]
            n104 = local read "TagNr"() -> (w224:enum16{"Tag 0", "Tag 1"})
            n105 = call "KH TURCK ETHERNETIP RFID UserCommand Array.vi"("BitArray"="Read", "UserCommand"=KH_TURCK_ETHERNETIP_TDef_Enum_RFID_User_Command."read", "TagNr"=w224) -> ("initialized array"=w221:bool[])  [unwired: 7 in, 1 out]
            n106 = local write "Read"(w221) -> ()
          }
          event "Write": Value Change {
            n107 = event-data() -> ()  [unwired: 1 in, 1 out]
            n108 = flat-sequence {
              tunnel: w231 -> [w234]
              tunnel: [w235] -> w229
              tunnel: ["TagNr"] -> w228
              tunnel: [w233] -> w227
              tunnel: [w258] -> w230
              tunnel: w229 -> [w258]
              tunnel: w228 -> [w257]
              tunnel: w227 -> [w256]
              frame #0 {
                n109 = call "KH TURCK ETHERNETIP RFID UserCommand Array.vi"("BitArray"="Write", "UserCommand"=KH_TURCK_ETHERNETIP_TDef_Enum_RFID_User_Command."write", "TagNr"="TagNr") -> ("index of element"=w233:i32, "initialized array"=w237:bool[])  [unwired: 7 in]
                n110 = local write "Write"(w237) -> ()
                n111 = case shown="\"Tag 1\"" "TagNr" {
                  tunnel: w233 -> [w245 w253]
                  tunnel: [w242 w252] -> w235
                  tunnel: w234 -> [w241 w251]
                  tunnel: w233 -> [w240 w248]
                  frame "Tag 0", Default {
                    n112 = case shown="1, Default" w245 {
                      tunnel: ["Write Kanal 0 Modul 2" "Write Kanal 0 Modul 1"] -> w244
                      frame 1, Default {
                        # "Modul 2"
                      }
                      frame 0 {
                        # "Modul 1"
                      }
                    }
                    n113 = call "KH TURCK ETHERNETIP FGlob RFID TAG0 AO.vi"("Nr Module"=w240, "Function"=KH_TURCK_TypeDefs_FGlob."Put one", "err in"=w241, "RFID one in"=w244) -> ("err out"=w242:errorcluster)  [unwired: 5 in, 2 out]
                  }
                  frame "Tag 1" {
                    n114 = case shown="0" w253 {
                      tunnel: ["Write Kanal 1 Modul 2" "Write Kanal 1 Modul 1"] -> w249
                      frame 1, Default {
                        # "Modul 2"
                      }
                      frame 0 {
                        # "Modul 1"
                      }
                    }
                    n115 = call "KH TURCK ETHERNETIP FGlob RFID TAG1 AO.vi"("Nr Module"=w248, "Function"=KH_TURCK_TypeDefs_FGlob."Put one", "err in"=w251, "RFID one in"=w249) -> ("err out"=w252:errorcluster)  [unwired: 5 in, 2 out]
                  }
                }
              }
              frame #1 {
                n116 = call "KH TURCK ETHERNETIP RFID WriteTag.vi"("Modul Nr"=w256, "TagNr"=w257) -> ()  [unwired: 10 in]
              }
            }
          }
          event "Inventory": Value Change {
            n117 = event-data() -> ()  [unwired: 1 in, 1 out]
            n118 = local read "TagNr"() -> (w262:enum16{"Tag 0", "Tag 1"})
            n119 = call "KH TURCK ETHERNETIP RFID UserCommand Array.vi"("BitArray"="Inventory", "UserCommand"=KH_TURCK_ETHERNETIP_TDef_Enum_RFID_User_Command."inventory", "TagNr"=w262) -> ("initialized array"=w259:bool[])  [unwired: 7 in, 1 out]
            n120 = local write "Inventory"(w259) -> ()
          }
          event "Reset message": Value Change {
            n121 = event-data() -> ()  [unwired: 1 in, 1 out]
            n122 = global read "KH TURCK ETHERNETIP RFID Global.vi" "RFID 0 LS Array"() -> (w268:T18[])
            n123 = global read "KH TURCK ETHERNETIP RFID Global.vi" "RFID 1 LS Array"() -> (w266:T18[])
            n124 = for {
              tunnel: [w278] -> w269 mode=indexing
              tunnel: w268 -> [w277] mode=indexing
              tunnel: [w276] -> w267 mode=indexing
              tunnel: w266 -> [w275] mode=indexing
              tunnel: [FALSE ("TimeoutReading")] -> w265 mode=indexing
              w274 = FALSE ("TimeoutReading")
              n125 = Bundle By Name(cluster=w277, "Timeout"=w274, "WritingFinished"=w274, "ReadingFinished"=w274) -> (w278:T18)
              n126 = Bundle By Name(cluster=w275, "Timeout"=w274, "WritingFinished"=w274, "ReadingFinished"=w274) -> (w276:T18)
            }
            n127 = global write "KH TURCK ETHERNETIP RFID Global.vi" "RFID 1 LS Array"(w267) -> ()
            n128 = global write "KH TURCK ETHERNETIP RFID Global.vi" "RFID 0 LS Array"(w269) -> ()
            n129 = global write "KH TURCK ETHERNETIP RFID Global.vi" "WritingSuccessfull0"(w265) -> ()
            n130 = global write "KH TURCK ETHERNETIP RFID Global.vi" "ErrorWriting0"(w265) -> ()
            n131 = global write "KH TURCK ETHERNETIP RFID Global.vi" "WritingSuccessfull1"(w265) -> ()
            n132 = global write "KH TURCK ETHERNETIP RFID Global.vi" "ErrorWriting1"(w265) -> ()
            n133 = local write "Reset message"(FALSE ("TimeoutWriting")) -> ()
          }
        }
      }
      n134 = while {
        i -> [w41]
        stop <- w38 stop-if-true
        n135 = Quotient & Remainder(x=w41, y=2) -> (x-y*floor(x/y)=w39:i32)  [unwired: 1 out]
        n136 = case shown="0" w39 {
          tunnel: [u16[] [0, 3] ("IOL Port 2") u16[] [0, 0] ("IOL Port 2")] -> w42
          frame 1, Default {
          }
          frame 0 {
          }
        }
        n137 = Bundle By Name(cluster=T14 {"IOL Port 1"=[0, 0], "IOL Port 2"=[0, 0], "IOL Port 3"=[0, 0], "IOL Port 4"=[0, 0]} ("Output_IOL 2"), "IOL Port 2"=w42) -> (w44:T14)
        n138 = local read "Exit"() -> (w38:bool)
        n139 = Wait Until Next ms Multiple(millisecond multiple=u32 3000) -> ()  [unwired: 1 out]
        n140 = local write "Output_IOL"(w44) -> ()
      }
      n141 = call "KH EthernetIP SetData.vi"("Function"="End", "error in"=w28) -> ("error out"=w32:errorcluster)  [unwired: 7 in, 2 out]
      n142 = call "KH EthernetIP GetData.vi"("Function"="End", "error in"=w35) -> ("error out"=w30:errorcluster)  [unwired: 8 in, 1 out]
      n143 = Merge Errors(w23, w32, w30, w26) -> (w31:errorcluster)
      n144 = call "KH EthernetIP OpenCloseConnection.vi"("Function"="Post", "error in"=w31) -> ("error out"=w25:errorcluster)  [unwired: 9 in]
    }
    frame Error {
      n145 = call <vilib>:"Simple Error Handler.vi"("error in (no error)"=w280) -> ("error out"=w279:errorcluster)  [unwired: 4 in, 4 out]
    }
  }
  n146 = flat-sequence {
    tunnel: w4 -> [w281]
    frame #0 {
      n147 = local write "Exit"(FALSE ("Exit")) -> ()
      "error out" <- w281
    }
  }
  n148 = disable-structure shown="Disabled" {
    frame Disabled {
      n149 = call "KH TURCK ETHERNETIP FGlob RFID TAG1 AO.vi"("Function"=KH_TURCK_TypeDefs_FGlob."Put one") -> ()  [unwired: 8 in, 3 out]
      n150 = call "KH TURCK ETHERNETIP FGlob RFID TAG0 AO.vi"("Function"=KH_TURCK_TypeDefs_FGlob."Put one") -> ()  [unwired: 8 in, 3 out]
      n151 = local read "Write Kanal 1 Modul 1"() -> ()  [unwired: 1 in]
      n152 = local read "Write Kanal 1 Modul 2"() -> ()  [unwired: 1 in]
      n153 = local read "Write Kanal 0 Modul 2"() -> ()  [unwired: 1 in]
    }
    frame Enabled {
    }
  }
